vi "Notification List entry.vi"(11 "Contacts in":string[](array[string])) -> (3 "Contacts out":string[](array[string]))   [LabVIEW 2012]
panel:
  in  "Cancel Button":bool
  in  "OK Button":bool
  in  "Contacts":string[](array[string])
  # "Send Notifications To:"
  # "Enter in an number of email addresses or\ncell phone numbers to receive warning\nemails and texts.\n\nexample how to send text message warnings..\n5551239876@vtext.com for verizon phones\n5551269876@txt.att.net for AT&T\n\nfor other providers contact the developer of \nthis application."
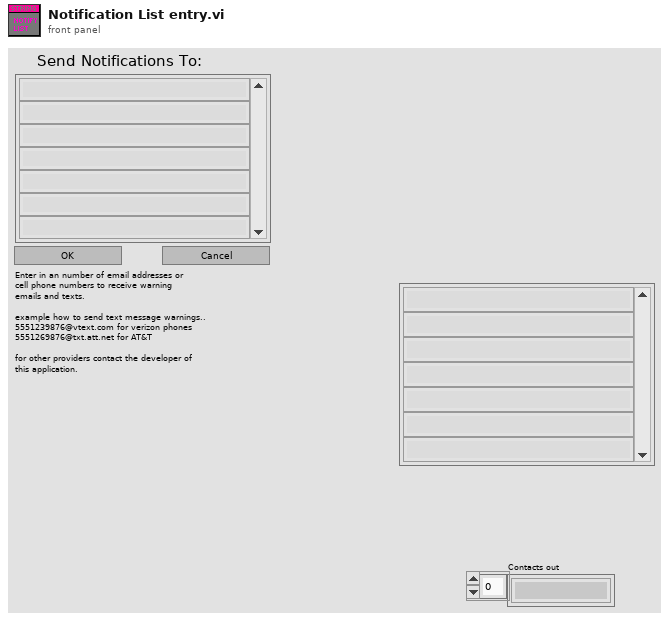
[diagram p1: front panel]
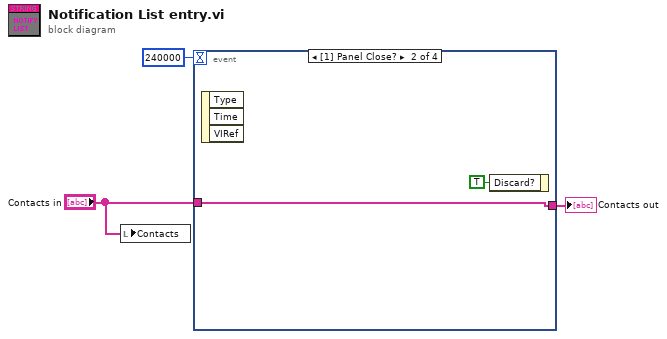
[diagram p0: block diagram]
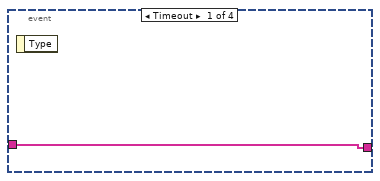
[diagram p2: hidden frame]
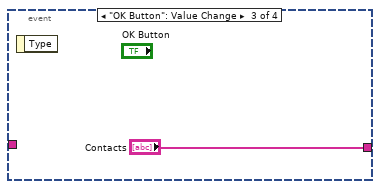
[diagram p3: hidden frame]
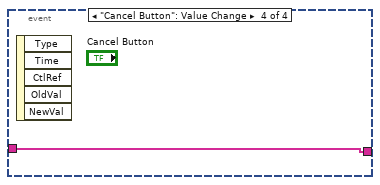
[diagram p4: hidden frame]
diagram:
  n1 = local write "Contacts"("Contacts in") -> ()
  n2 = event shown="[1] Panel Close?" {
    selector: _ -> [_ _ _ _]
    dyn-events: _ -> [_ _ _ _]
    timeout: 240000 -> [_ _ _ _]
    tunnel: "Contacts in" -> [w4 w6 _ w8]
    tunnel: [w4 w6 "Contacts" w8] -> w2
    event Timeout {
      n3 = event-data() -> ()  [unwired: 1 in, 1 out]
    }
    event Panel Close? {
      n4 = event-data() -> ()  [unwired: 1 in, 3 out]
      n5 = event-data("Discard?"=TRUE) -> ()  [unwired: 1 in, 1 out]
    }
    event "OK Button": Value Change {
      n6 = event-data() -> ()  [unwired: 1 in, 1 out]
    }
    event "Cancel Button": Value Change {
      n7 = event-data() -> ()  [unwired: 1 in, 5 out]
    }
  }
  "Contacts out" <- w2
